vi "tasksink.vi"(0 "task_nbr":i32) -> ()   [LabVIEW 2014]
uses:
  <vilib>/addons/zeromq/socket_type.ctl
  <vilib>/addons/zeromq/zmq_context.lvclass
  <vilib>/addons/zeromq/zeromq.lvlib
  <vilib>/addons/zeromq/zmq_socket.lvclass
panel:
  out "data 2":string
  out "data":string
  out "Using Time: %d ms":dbl
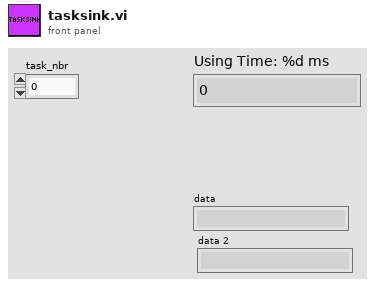
[diagram p1: front panel]
types:
  T1 = typedef "zeromq.lvlib/socket_type.ctl" = enum8{"ZMQ_PAIR", "ZMQ_PUB", "ZMQ_SUB", "ZMQ_REQ", "ZMQ_REP", "ZMQ_DEALER", "ZMQ_ROUTER", "ZMQ_PULL", "ZMQ_PUSH", "ZMQ_XPUB", "ZMQ_XSUB"}
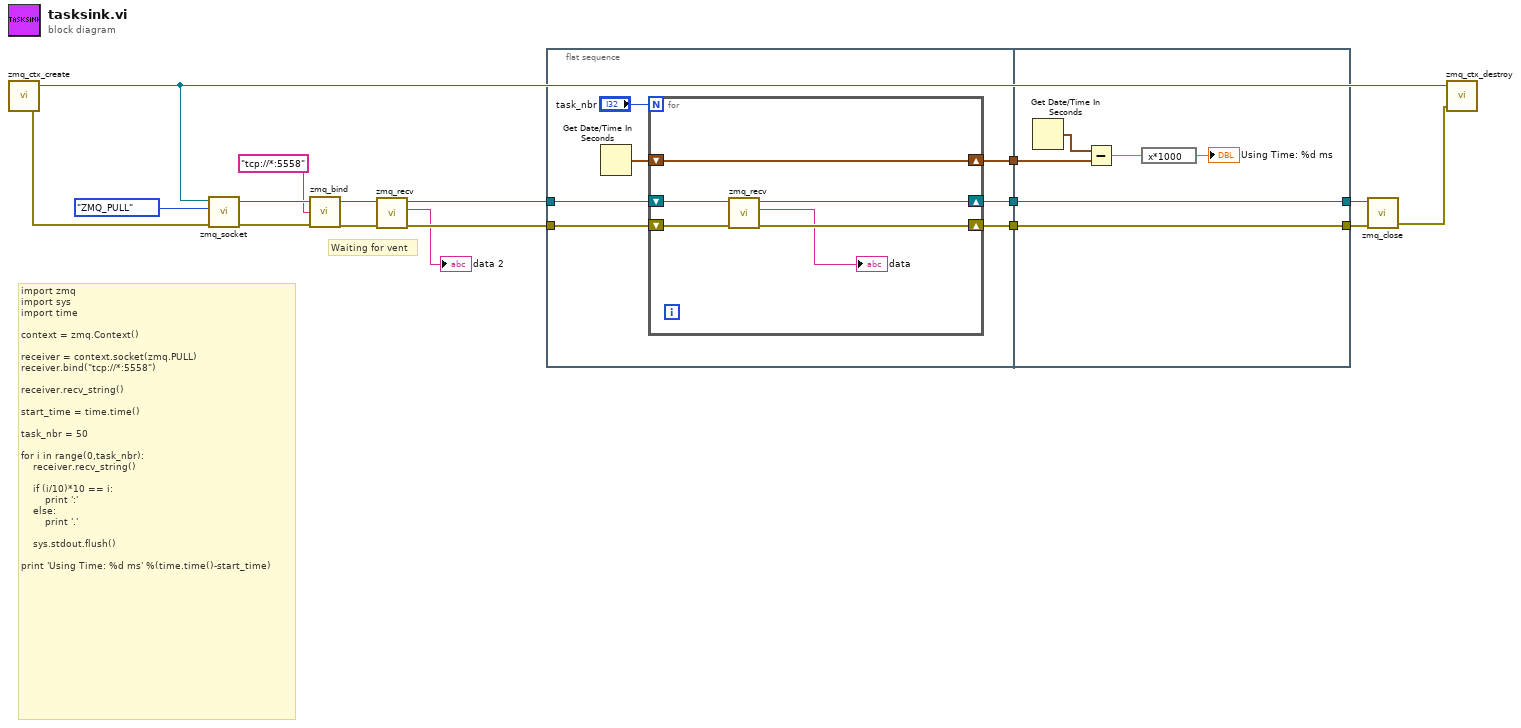
[diagram p0: block diagram]
diagram:
  # "Waiting for vent"
  # "import zmq\nimport sys\nimport time\n\ncontext = zmq.Context()\n\nreceiver = context.socket(zmq.PULL)\nreceiver.bind(\"tcp://*:5558\")\n\nreceiver.recv_string()\n\nstart_time = time.time()\n\ntask_nbr = 50\n\nfor i in range(0,task_nbr):\n    receiver.recv_string()\n\n    if (i/10)*10 == i:\n        print ':'\n    else:\n        print '.'\n\n    sys.stdout.flush()\n\nprint 'Using Time: %d ms' %(time.time()-start_time)"
  n1 = call <vilib>:"zmq_ctx_create.vi"() -> ("error out"=w16:errorcluster, "context out"=w15:refnum<class "zmq_context.lvclass">)  [unwired: 4 in]
  n2 = call <vilib>:"zmq_socket.vi"("error in"=w16, "socket type"=socket_type."ZMQ_PULL", "context in"=w15) -> ("error out"=w13:errorcluster, "socket out"=w14:refnum<class "zmq_socket.lvclass">)  [unwired: 2 in, 1 out]
  n3 = call <vilib>:"zmq_bind.vi"("error in"=w13, "endpoint"="tcp://*:5558", "socket in"=w14) -> ("error out"=w9:errorcluster, "socket out"=w10:refnum<class "zmq_socket.lvclass">)  [unwired: 1 in]
  n4 = call <vilib>:"zmq_recv.vi"("error in"=w9, "socket in"=w10) -> ("error out"=w8:errorcluster, "data"=→"data 2":string, "socket out"=w7:refnum<class "zmq_socket.lvclass">)  [unwired: 3 in, 2 out]
  n5 = flat-sequence {
    tunnel: w8 -> [w24]
    tunnel: w7 -> [w23]
    tunnel: [w22] -> w4
    tunnel: [w21] -> w3
    tunnel: [w18] -> w2
    tunnel: [w35] -> w5
    tunnel: [w36] -> w6
    tunnel: w4 -> [w36]
    tunnel: w3 -> [w35]
    tunnel: w2 -> [w33]
    frame #0 {
      n6 = Get Date/Time In Seconds() -> (seconds since 1Jan1904=w20:timestamp)
      n7 = for {
        N: "task_nbr" -> [_]
        shift-right: [w27] -> w21
        shift-left: w24 -> [w30]
        shift-right: [w28] -> w22
        shift-left: w23 -> [w29]
        shift-right: [w26] -> w18
        shift-left: w20 -> [w26]
        n8 = call <vilib>:"zmq_recv.vi"("error in"=w30, "socket in"=w29) -> ("error out"=w27:errorcluster, "data"=→"data":string, "socket out"=w28:refnum<class "zmq_socket.lvclass">)  [unwired: 3 in, 2 out]
      }
    }
    frame #1 {
      n9 = Get Date/Time In Seconds() -> (seconds since 1Jan1904=w34:timestamp)
      n10 = Subtract(x=w34, y=w33) -> (x-y=w32:dbl)
      n11 = expression code="x*1000"(w32) -> (→"Using Time: %d ms":dbl)
    }
  }
  n12 = call <vilib>:"zmq_close.vi"("error in"=w5, "socket"=w6) -> ("error out"=w11:errorcluster)  [unwired: 3 in]
  n13 = call <vilib>:"zmq_ctx_destroy.vi"("error in"=w11, "context in"=w15) -> ()  [unwired: 3 in, 1 out]
